vi "getHWConfig.vi"(8 "error in (no error)":errorcluster, 11 "HWConfiguration in":refnum<class "HWConfiguration.lvclass">) -> (0 "error out":errorcluster, 3 "HWConfiguration out":refnum<class "HWConfiguration.lvclass">)   [LabVIEW 2009, in "Hardware.lvlib" / "HWControllers.lvlib" / "HWConfiguration.lvclass"]
uses:
  HWConfiguration.lvclass
  HWConfiguration.lvclass/HWConfiguration.ctl
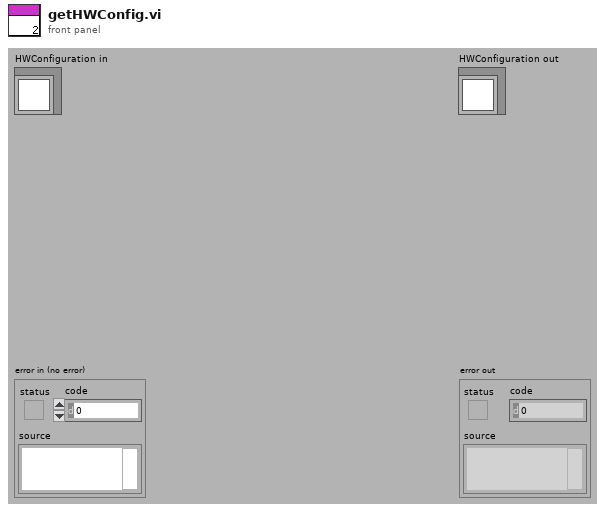
[diagram p1: front panel]
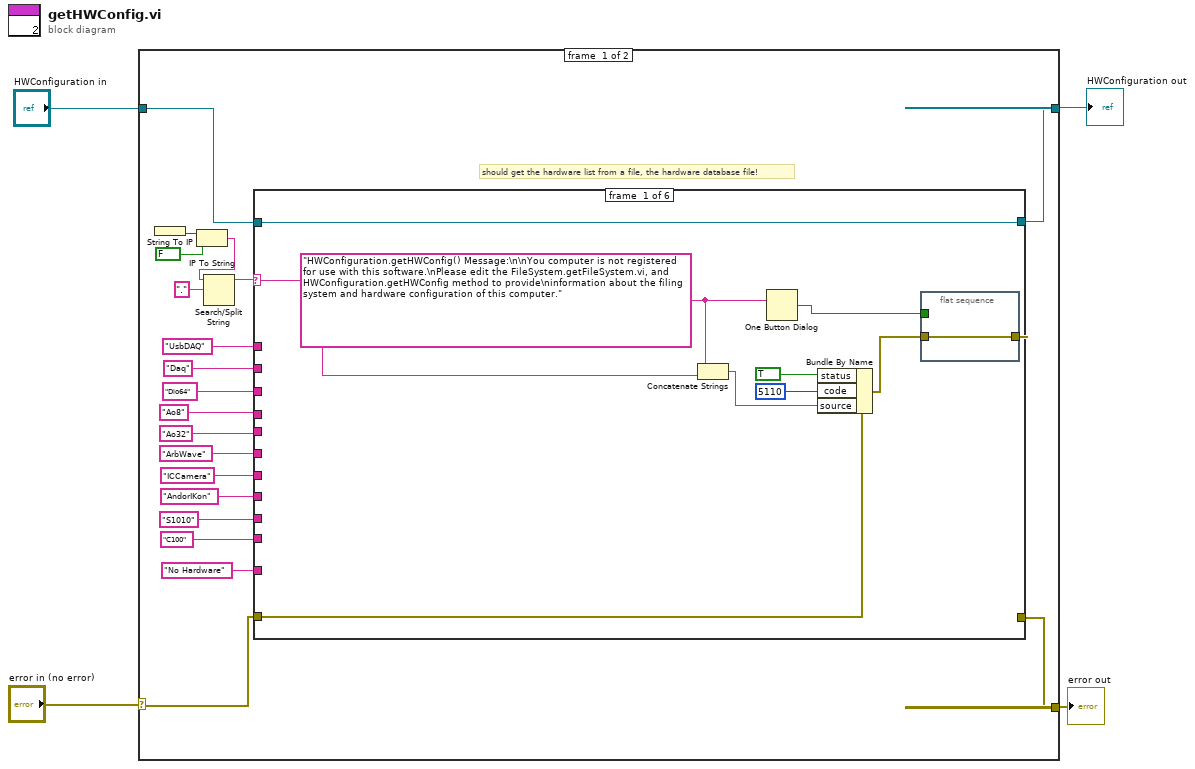
[diagram p0: block diagram]
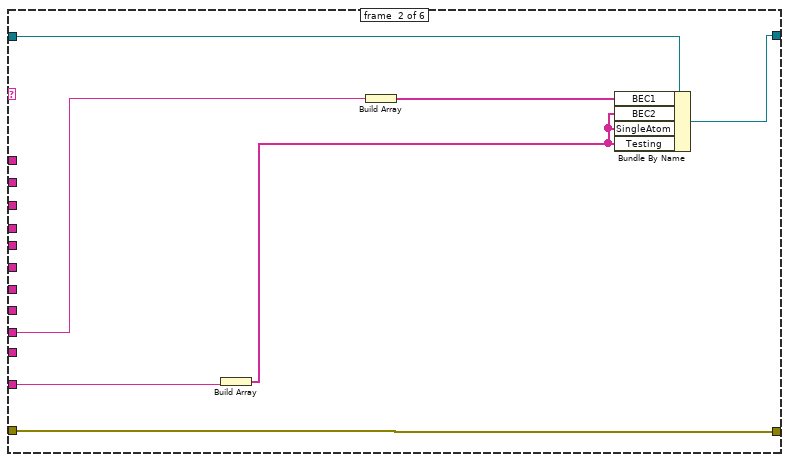
[diagram p2: hidden frame]
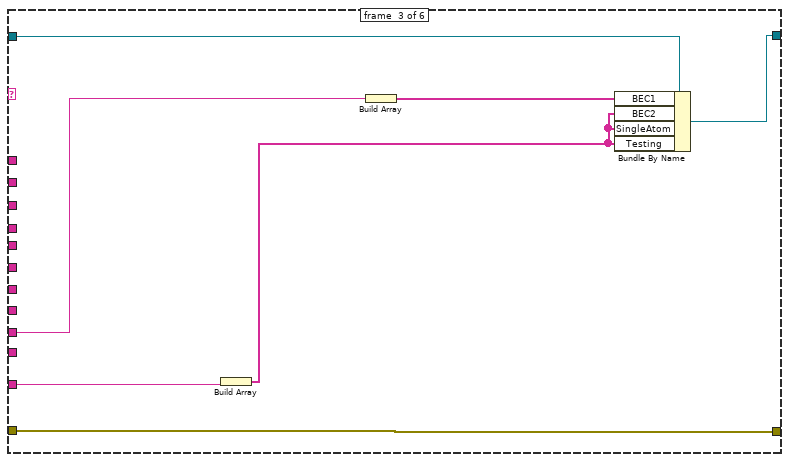
[diagram p3: hidden frame]
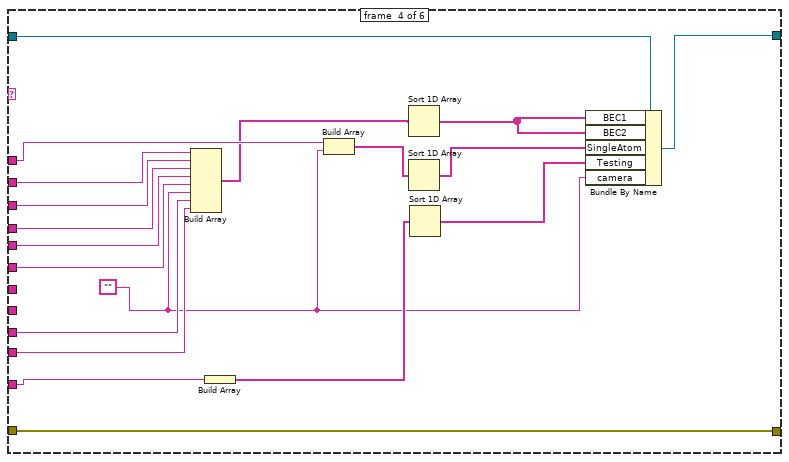
[diagram p4: hidden frame]
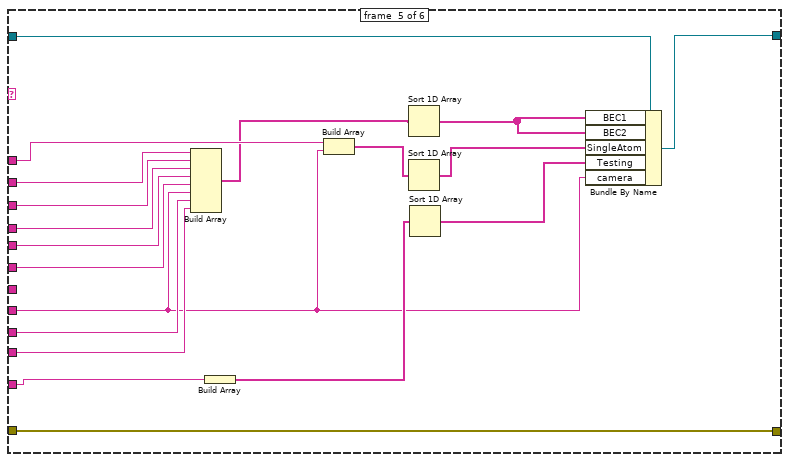
[diagram p5: hidden frame]
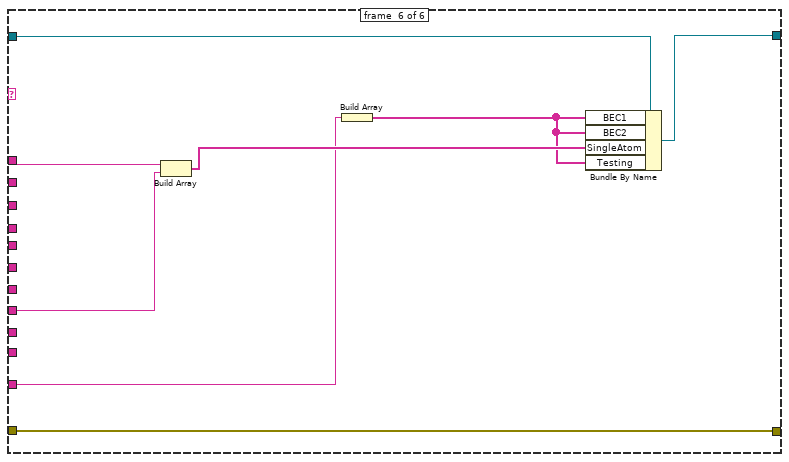
[diagram p6: hidden frame]
diagram:
  n1 = case shown="No Error" "error in (no error)" {
    selector: "error in (no error)" -> [w19 w97]
    tunnel: [w16 w97] -> w3
    tunnel: [w17 w96] -> w1
    tunnel: "HWConfiguration in" -> [w18 w96]
    frame #0 {
      # "should get the hardware list from a file, the hardware database file!"
      n2 = String To IP() -> (0:w23:u32)  [unwired: 1 in]
      n3 = IP To String(1:FALSE, 2:w23) -> (0:w21:string)
      n4 = Search/Split String(string=w21, search string/char (-)=".") -> (substring before match=w20:string)  [unwired: 1 in, 2 out]
      n5 = case shown="\"becartemis\", Default" w20 {
        selector: w20 -> [w28 _ _ _ _ _]
        tunnel: w18 -> [w25 w41 w48 w67 w86 w94]
        tunnel: [w25 w40 w47 w66 w85 w93] -> w17
        tunnel: w19 -> [w26 w42 w49 w68 w87 w95]
        tunnel: [w31 w42 w49 w68 w87 w95] -> w16
        tunnel: "UsbDAQ" -> [_ _ _ w58 w77 w92]
        tunnel: "Daq" -> [_ _ _ w65 w84 _]
        tunnel: "Dio64" -> [_ _ _ w51 w70 _]
        tunnel: "Ao8" -> [_ _ _ w64 w83 _]
        tunnel: "Ao32" -> [_ _ _ w63 w82 _]
        tunnel: "ArbWave" -> [_ _ _ w62 w81 _]
        tunnel: "ICCamera" -> [_ _ _ _ _ _]
        tunnel: "AndorIKon" -> [_ _ _ _ w69 w91]
        tunnel: "S1010" -> [_ w37 w44 w61 w80 _]
        tunnel: "C100" -> [_ _ _ w60 w79 _]
        tunnel: "No Hardware" -> [_ w39 w46 w59 w78 w88]
        frame #0 {
          w29 = "HWConfiguration.getHWConfig() Message:\n\nYou computer is not registered for use with this software.\nPlease edit the FileSystem.getFileSystem.vi, and HWConfiguration.getHWConfig method to provide\ninformation about the filing system and hardware configuration of this computer."
          n6 = Concatenate Strings(w29, w28) -> (w27:string)
          n7 = One Button Dialog(message=w29) -> (true=w30:bool)  [unwired: 1 in]
          n8 = Bundle By Name(cluster=w26, "status"=TRUE, "code"=5110, "source"=w27) -> (w32:errorcluster)
          n9 = flat-sequence {
            tunnel: w32 -> [w35]
            tunnel: [w35] -> w31
            tunnel: w30 -> [_]
            frame #0 {
            }
          }
        }
        frame #1 {
          n10 = Build Array(w39) -> (w38:string[])
          n11 = Build Array(w37) -> (w36:string[])
          n12 = Bundle By Name(cluster=w41, "BEC1"=w36, "BEC2"=w38, "SingleAtom"=w38, "Testing"=w38) -> (w40:refnum<class "HWConfiguration.lvclass">)
        }
        frame #2 {
          n13 = Build Array(w46) -> (w45:string[])
          n14 = Build Array(w44) -> (w43:string[])
          n15 = Bundle By Name(cluster=w48, "BEC1"=w43, "BEC2"=w45, "SingleAtom"=w45, "Testing"=w45) -> (w47:refnum<class "HWConfiguration.lvclass">)
        }
        frame #3 {
          w50 = ""
          n16 = Build Array(w65, w51, w64, w63, w62, w50, w61, w60) -> (w57:string[])
          n17 = Build Array(w59) -> (w53:string[])
          n18 = Build Array(w58, w50) -> (w55:string[])
          n19 = Sort 1D Array(array=w57) -> (sorted array=w56:string[])
          n20 = Sort 1D Array(array=w55) -> (sorted array=w54:string[])
          n21 = Sort 1D Array(array=w53) -> (sorted array=w52:string[])
          n22 = Bundle By Name(cluster=w67, "BEC1"=w56, "BEC2"=w56, "SingleAtom"=w54, "Testing"=w52, "camera"=w50) -> (w66:refnum<class "HWConfiguration.lvclass">)
        }
        frame #4 {
          n23 = Build Array(w84, w70, w83, w82, w81, w69, w80, w79) -> (w76:string[])
          n24 = Build Array(w78) -> (w72:string[])
          n25 = Build Array(w77, w69) -> (w74:string[])
          n26 = Sort 1D Array(array=w76) -> (sorted array=w75:string[])
          n27 = Sort 1D Array(array=w74) -> (sorted array=w73:string[])
          n28 = Sort 1D Array(array=w72) -> (sorted array=w71:string[])
          n29 = Bundle By Name(cluster=w86, "BEC1"=w75, "BEC2"=w75, "SingleAtom"=w73, "Testing"=w71, "camera"=w69) -> (w85:refnum<class "HWConfiguration.lvclass">)
        }
        frame #5 {
          n30 = Build Array(w92, w91) -> (w90:string[])
          n31 = Build Array(w88) -> (w89:string[])
          n32 = Bundle By Name(cluster=w94, "BEC1"=w89, "BEC2"=w89, "SingleAtom"=w90, "Testing"=w89) -> (w93:refnum<class "HWConfiguration.lvclass">)
        }
      }
    }
    frame #1 {
    }
  }
  "error out" <- w3
  "HWConfiguration out" <- w1
